vi "Create.vi"(8 "error in (no error)":errorcluster, 10 "VI":refnum<vi>) -> (0 "error out":errorcluster, 3 "Call Out":refnum<class "VI Call.lvclass">)   [LabVIEW 2020, in "VI Call.lvclass"]
uses:
  VI Call.lvclass
  VI Call.lvclass/VI Call.ctl
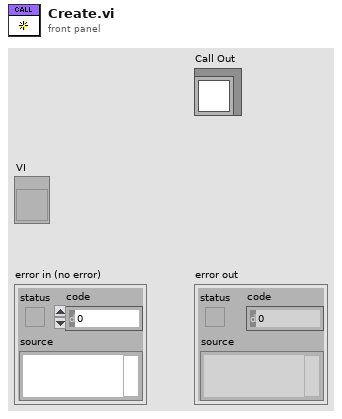
[diagram p1: front panel]
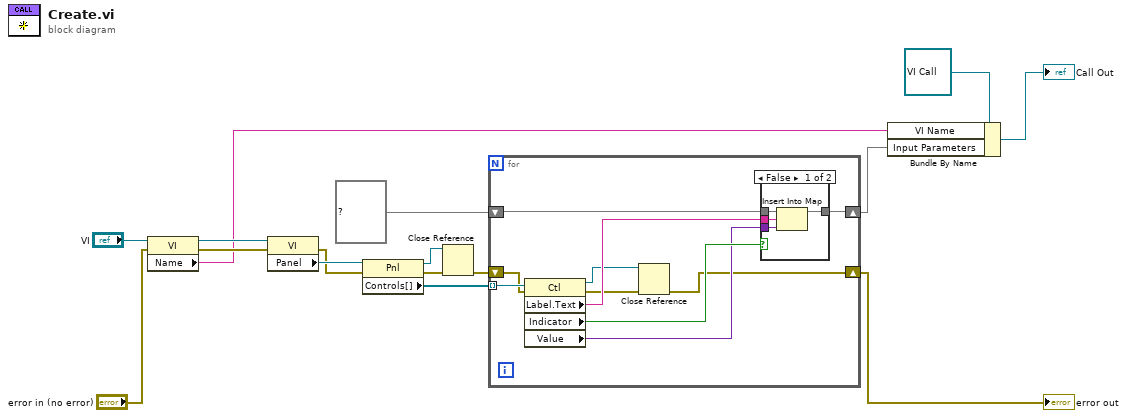
[diagram p0: block diagram]
diagram:
  n1 = property class="VI"(reference="VI", error in="error in (no error)") -> (reference out=w15:refnum<vi>, error out=w10:errorcluster, "Name"=w3:string)
  n2 = property class="VI"(reference=w15, error in=w10) -> (error out=w9:errorcluster, "Panel"=w14:refnum<vi>)  [unwired: 1 out]
  n3 = property class="Pnl"(reference=w14, error in=w9) -> (reference out=w1:refnum<vi>, error out=w8:errorcluster, "Controls[]"=w13:refnum<vi>[])
  n4 = Close Reference(reference=w1, error in (no error)=w8) -> (error out=w2:errorcluster)
  n5 = for {
    tunnel: w13 -> [w26] mode=indexing
    shift-right: [w24] -> w4
    shift-left: map{string, variant} {} ("map") -> [w25]
    shift-right: [w18] -> w7
    shift-left: w2 -> [w20]
    n6 = property class="Ctl"(reference=w26, error in=w20) -> (reference out=w17:refnum<vi>, error out=w19:errorcluster, "Label.Text"=w23:string, "Indicator"=w22:bool, "Value"=w21:variant)
    n7 = Close Reference(reference=w17, error in (no error)=w19) -> (error out=w18:errorcluster)
    n8 = case shown="False" w22 {
      tunnel: w25 -> [w30 w31]
      tunnel: [w29 w31] -> w24
      tunnel: w23 -> [w28 _]
      tunnel: w21 -> [w27 _]
      frame False {
        n9 = Insert Into Map(map in=w30, key=w28, value=w27) -> (map out=w29:map{string, variant})  [unwired: 2 out]
      }
      frame True {
      }
    }
  }
  "error out" <- w7
  n10 = Bundle By Name(cluster=refnum<class "VI Call.lvclass"> refnum ("Call"), "VI Name"=w3, "Input Parameters"=w4) -> (→"Call Out":refnum<class "VI Call.lvclass">)
